vi "niDTS WLAN UTIL Format MAC Address.vi"(8 "error in (no error)":errorcluster, 11 "MAC Address In":string) -> (0 "error out":errorcluster, 3 "MAC Address Out":string)   [LabVIEW 2015, in "niDTS WLAN.lvlib"]
uses:
  niDTS WLAN.lvlib
  Dependencies/__Error Cluster From Error Code.vi
  Dependencies/__Error Ring.xnode
  Dependencies/__Match Regular Expression.xnode
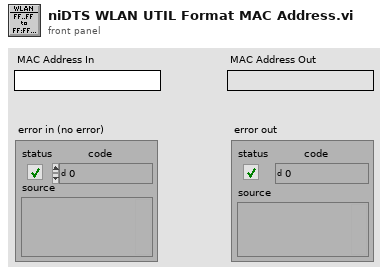
[diagram p1: front panel]
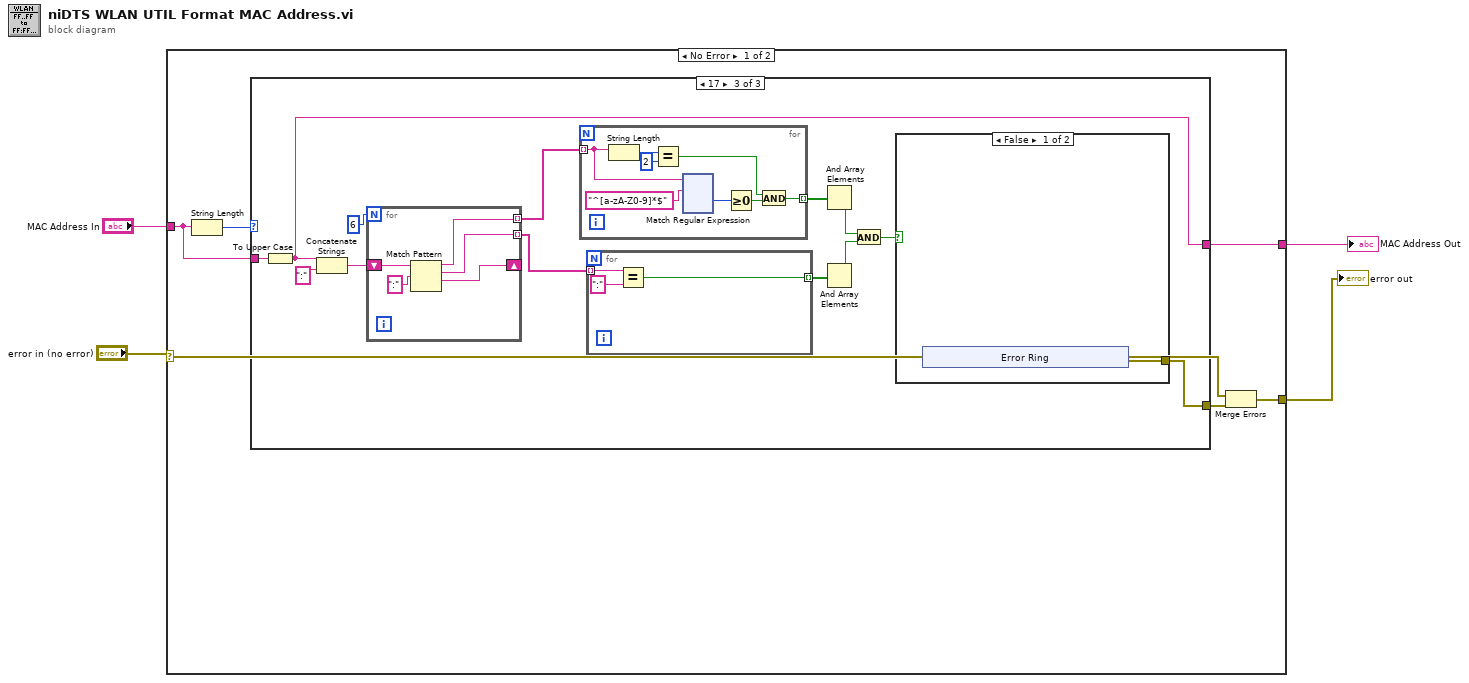
[diagram p0: block diagram]
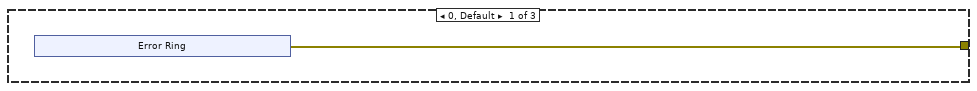
[diagram p2: hidden frame]
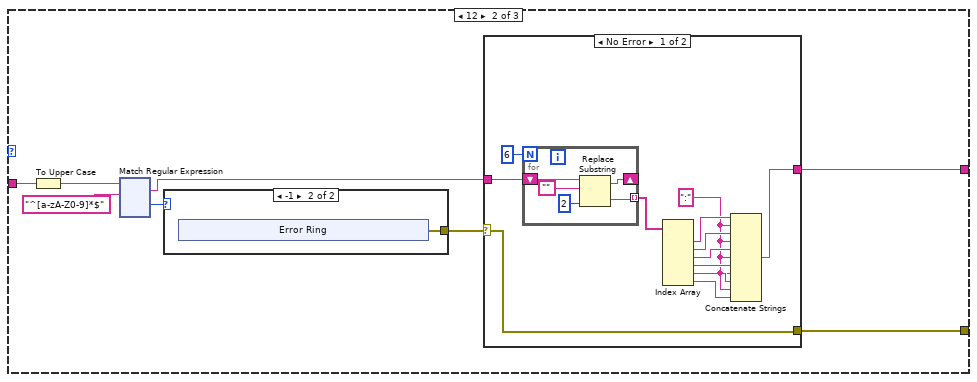
[diagram p3: hidden frame]
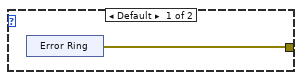
[diagram p5: hidden frame]
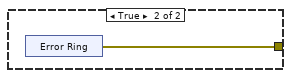
[diagram p6: hidden frame]
diagram:
  n1 = case shown="No Error" "error in (no error)" {
    selector: "error in (no error)" -> [w8 _]
    tunnel: "MAC Address In" -> [w6 w317]
    tunnel: [w7 _] -> w2
    tunnel: [w5 w317] -> w1
    frame No Error {
      n2 = String Length(string=w6) -> (length=w10:i32)
      n3 = case shown="17" w10 {
        tunnel: [w11 w19 w167] -> w9
        tunnel: w6 -> [_ w24 w178]
        tunnel: [_ w17 w166] -> w5
        frame 0, Default {
          n4 = xnode "Error Ring"() -> ("error out"=w11:errorcluster)
        }
        frame 12 {
          n5 = To Upper Case(1:w24) -> (0:w22:string)
          n6 = xnode "Match Regular Expression"("input string"=w22, "regular expression"="^[a-zA-Z0-9]*$") -> ("whole match"=w18:string, "offset past match"=w21:i32)  [unwired: 4 in, 3 out]
          n7 = case shown="-1" w21 {
            tunnel: [w44 w46] -> w20
            frame Default {
              n8 = xnode "Error Ring"() -> ("error out"=w44:errorcluster)
            }
            frame -1 {
              n9 = xnode "Error Ring"() -> ("error out"=w46:errorcluster)
            }
          }
          n10 = case shown="No Error" w20 {
            selector: w20 -> [w36 w43]
            tunnel: [w36 w43] -> w19
            tunnel: w18 -> [w34 w42]
            tunnel: [w25 w42] -> w17
            frame No Error {
              w27 = ":"
              n11 = for {
                N: 6 -> [_]
                shift-right: [w38] -> _
                shift-left: w34 -> [w41]
                tunnel: [w37] -> w33 mode=indexing
                n12 = Replace Substring(2:2 ("length (len. of substring)"), 4:"", 5:w41) -> (0:w37:string, 1:w38:string)  [unwired: 1 in]
              }
              n13 = Index Array(array=w33) -> (element #1=w32:string, element #2=w31:string, element #3=w30:string, element #4=w29:string, element #5=w28:string, element #6=w26:string)  [unwired: 6 in]
              n14 = Concatenate Strings(w32, w27, w31, w27, w30, w27, w29, w27, w28, w27, w26) -> (w25:string)
            }
            frame Error {
            }
          }
        }
        frame 17 {
          n15 = To Upper Case(1:w178) -> (0:w166:string)
          n16 = Concatenate Strings(w166, ":") -> (w176:string)
          n17 = for {
            N: 6 -> [_]
            shift-right: [w312] -> _
            shift-left: w176 -> [w316]
            tunnel: [w314] -> w174 mode=indexing
            tunnel: [w313] -> w172 mode=indexing
            n18 = Match Pattern(string=w316, regular expression=":") -> (before substring=w314:string, match substring=w313:string, after substring=w312:string)  [unwired: 1 in, 1 out]
          }
          n19 = for {
            tunnel: w174 -> [w194] mode=indexing
            tunnel: [w190] -> w173 mode=indexing
            n20 = String Length(string=w194) -> (length=w197:i32)
            n21 = Equal?(x=w197, y=2) -> (x = y?=w191:bool)
            n22 = xnode "Match Regular Expression"("input string"=w194, "regular expression"="^[a-zA-Z0-9]*$") -> ("offset past match"=w193:i32)  [unwired: 4 in, 4 out]
            n23 = Greater Or Equal To 0?(x=w193) -> (x >= 0?=w192:bool)
            n24 = And(x=w191, y=w192) -> (x .and. y?=w190:bool)
          }
          n25 = for {
            tunnel: w172 -> [w189] mode=indexing
            tunnel: [w187] -> w171 mode=indexing
            n26 = Equal?(x=w189, y=":") -> (x = y?=w187:bool)
          }
          n27 = And Array Elements(Boolean array=w173) -> (logical AND=w169:bool)
          n28 = And Array Elements(Boolean array=w171) -> (logical AND=w170:bool)
          n29 = And(x=w169, y=w170) -> (x .and. y?=w168:bool)
          n30 = case shown="False" w168 {
            tunnel: [w179 w185] -> w167
            frame False {
              n31 = xnode "Error Ring"() -> ("error out"=w179:errorcluster)
            }
            frame True {
              n32 = xnode "Error Ring"() -> ("error out"=w185:errorcluster)
            }
          }
        }
      }
      n33 = Merge Errors(w8, w9) -> (w7:errorcluster)
    }
    frame Error {
    }
  }
  "MAC Address Out" <- w1
  "error out" <- w2
